vi "BackTracking.vi"(11 "Pontos":dbl[][](array[numeric])) -> (2 "element":dbl, 3 "Path":dbl[][](array[numeric]))   [LabVIEW 2018]
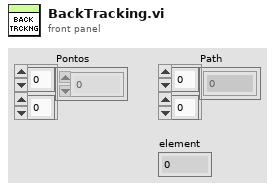
[diagram p1: front panel]
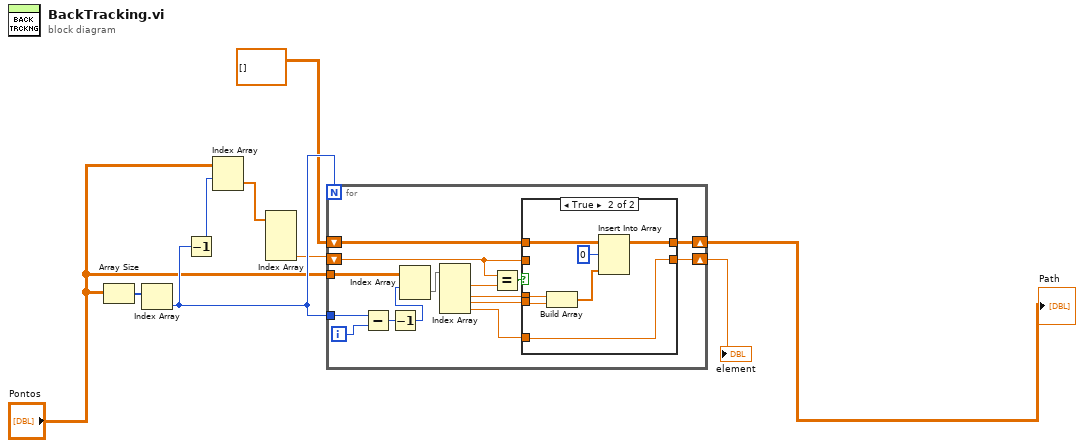
[diagram p0: block diagram]
diagram:
  n1 = Array Size(array="Pontos") -> (size(s)=w1:i32[])
  n2 = Index Array(array=w1) -> (element=w8:i32)  [unwired: 1 in]
  n3 = Decrement(x=w8) -> (x-1=w6:i32)
  n4 = Index Array(array="Pontos", index (row)=w6) -> (element=w4:dbl[])  [unwired: 1 in]
  n5 = Index Array(array=w4) -> (element #4=w5:dbl)  [unwired: 4 in, 3 out]
  n6 = for {
    N: w8 -> [_]
    shift-right: [w20] -> w9
    shift-left: dbl[][] [] ("Path") -> [w21]
    tunnel: w8 -> [w19]
    tunnel: "Pontos" -> [w17]
    shift-right: [w14] -> w2
    shift-left: w5 -> [w12]
    i -> [w18]
    n7 = Subtract(x=w19, y=w18) -> (x-y=w11:i32)
    n8 = Decrement(x=w11) -> (x-1=w10:i32)
    n9 = Index Array(array=w17, index (row)=w10) -> (element=w16:dbl[])  [unwired: 1 in]
    n10 = Index Array(array=w16) -> (element #1=w15:dbl, element #2=w23:dbl, element #3=w22:dbl, element #4=w13:dbl)  [unwired: 4 in]
    n11 = Equal?(x=w12, y=w15) -> (x = y?=w24:bool)
    n12 = case shown="True" w24 {
      tunnel: w23 -> [_ w33]
      tunnel: w22 -> [_ w32]
      tunnel: w21 -> [w26 w31]
      tunnel: [w26 w29] -> w20
      tunnel: [w25 w28] -> w14
      tunnel: w13 -> [_ w28]
      tunnel: w12 -> [w25 _]
      frame False {
      }
      frame True {
        n13 = Build Array(w33, w32) -> (w30:dbl[])
        n14 = Insert Into Array(array=w31, index (row)=0, new element=w30) -> (w29:dbl[][])  [unwired: 1 in]
      }
    }
  }
  "element" <- w2
  "Path" <- w9
